vi "Create and Load SensorLUT Dictionary.vi"(8 "error in (no error)":errorcluster, 11 "Main in":refnum<class "Main.lvclass">) -> (0 "error out":errorcluster, 3 "Main out":refnum<class "Main.lvclass">)   [LabVIEW 2019, in "Main.lvclass"]
uses:
  Main.lvclass
  Main.lvclass/Main.ctl
  Common/DataTypes/Sensor LUT--cluster.ctl
  Common/DataTypes/Sensor database record--cluster.ctl
  Common/DataTypes/Sensor ranges--cluster.ctl
  Accessors/Set CurrSensor Record.vi
  Accessors/Get Settings.vi
  <userlib>/_OpenG.lib/file/file.llb/File Exists - Scalar__ogtk.vi
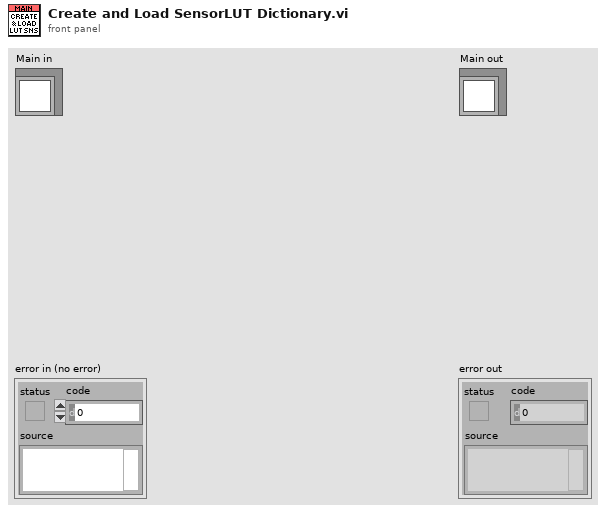
[diagram p1: front panel]
types:
  T1 = typedef "Main.lvclass/Settings--cluster.ctl" = cluster{"Simulation":bool, "Signal scaling":T2[], "ESR scaling":T3[], "num readings to average":i32[], "ESR alarm threshhold (%)":i32[], "UseDummyVrms":bool, "Dummy Vrms":dbl, "Inverter Database File":path, "default Inverter (name)":string[], "Minimum Current Threshold ":dbl[], "Sensors Database File":path, "default Sensors (name)":string[]}
  T2 = typedef "Main.lvclass/Gain control.ctl" = cluster{"Iin ripple gain":dbl, "Iout ripple gain":dbl, "Iout 60Hz gain ":dbl, "Vout 60Hz gain ":dbl, "Iin ripple offest":dbl, "Iout ripple offset":dbl, "Iout 60Hz offset":dbl, "Vout 60Hz offset":dbl}
  T3 = typedef "Main.lvclass/ESR scaling--cluster.ctl" = cluster{"Gain":dbl, "Offset":dbl}
  T4 = typedef "Sensor LUT--cluster.ctl" = T5[]
  T5 = typedef "Sensor database record--cluster.ctl" = cluster{"name":string, "last updated":timestamp, "manufacturer":string, "model":string, "Sensitivity index":dbl, "Sensor Ranges":T6}
  T6 = typedef "Sensor ranges--cluster.ctl" = cluster{"Max.VOut.RMS (V)":dbl, "Max.Out.Peak (V)":dbl, "Sensitivity (mV/A)":dbl, "Max.IOut.RMS(A)":dbl, "Min.IOut.RMS(A)":dbl}
  T7 = typedef "TD Dynamic CVT DVR--ref.ctl" = refnum<data-value>
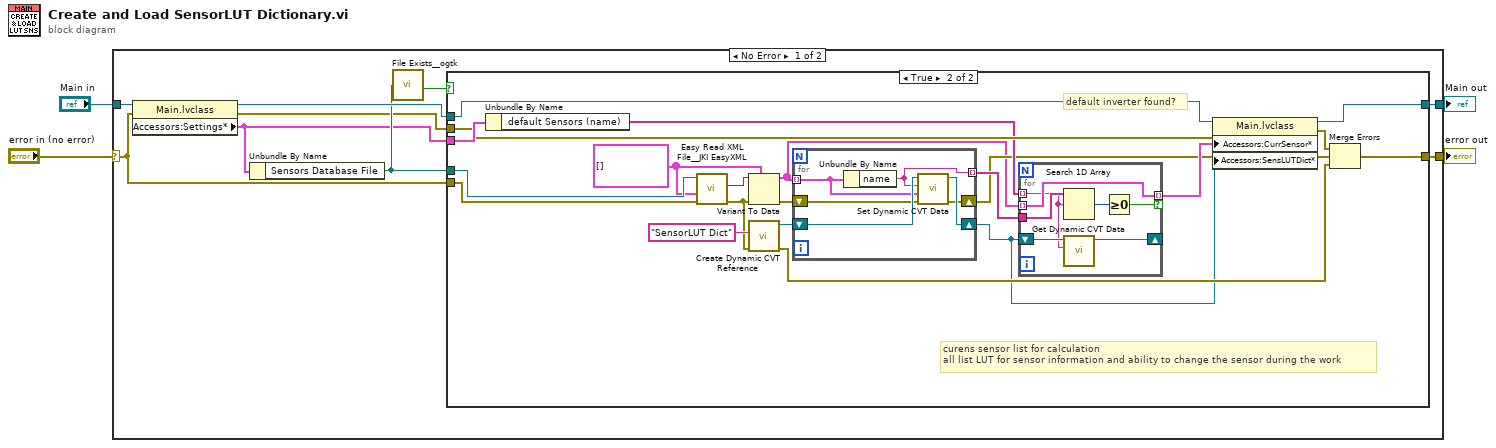
[diagram p0: block diagram]
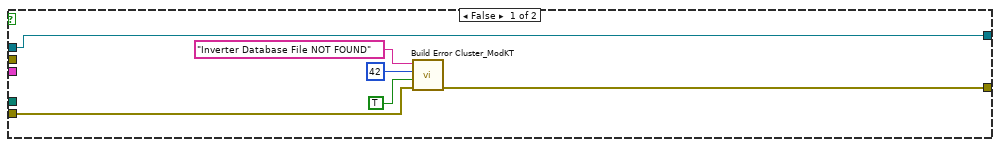
[diagram p2: hidden frame]
diagram:
  n1 = case shown="No Error" "error in (no error)" {
    selector: "error in (no error)" -> [w11 w55]
    tunnel: [w12 w55] -> w1
    tunnel: [w10 w54] -> w2
    tunnel: "Main in" -> [w13 w54]
    frame No Error {
      n2 = property class="Main.lvclass"(reference=w13, error in=w11) -> (reference out=w9:refnum<class "Main.lvclass">, error out=w5:errorcluster, "Accessors:Settings*"=w6:T1)
      n3 = Unbundle By Name(w6) -> ("Sensors Database File"=w8:path)
      n4 = call-poly <userlib>:"File Exists__ogtk.vi"("file path"=w8) -> ("exists"=w7:bool)  [unwired: 6 in, 1 out]
      n5 = case shown="True" w7 {
        tunnel: [w18 w28] -> w12
        tunnel: w8 -> [_ w38]
        tunnel: w11 -> [w17 w37]
        tunnel: [w19 w30] -> w10
        tunnel: w9 -> [w19 w36]
        tunnel: w6 -> [_ w31]
        tunnel: w5 -> [_ w29]
        frame False {
          n6 = call <vilib>:"Build Error Cluster_ModKT .vi"("Prepend String (\"\")"="Inverter Database File NOT FOUND" ("Prepend String (\"\")"), "code"=42, "error? (F)"=TRUE, "error in (no error)"=w17) -> ("error out"=w18:errorcluster)  [unwired: 3 in, 1 out]
        }
        frame True {
          w21 = T4 [] ("Sensor Records")
          # "curens sensor list for calculation\nall list LUT for sensor information and ability to change the sensor during the work"
          # "default inverter found?"
          n7 = Unbundle By Name(w31) -> ("default Sensors (name)"=w25:string[])
          n8 = call <vilib>:"Easy Read XML File__JKI EasyXML.vi"("error in (no error)"=w37, "LabVIEW Data (Type)"=w21, "XML File Path"=w38) -> ("error out"=w35:errorcluster, "LabVIEW Data"=w34:variant)  [unwired: 6 in, 1 out]
          n9 = Variant To Data(error in=w35, type=w21, Variant=w34) -> (data=w22:T4, error out=w33:errorcluster)
          n10 = call <vilib>:"Create Dynamic CVT Reference.vi"("error in (no error)"=w35, "DictName"="SensorLUT Dict") -> ("error out"=w40:errorcluster, "dCVT DVR out"=w32:T7)  [unwired: 8 in]
          n11 = for {
            tunnel: w22 -> [w49] mode=indexing
            shift-right: [w50] -> w23
            shift-left: w33 -> [w51]
            shift-right: [w52] -> w20
            shift-left: w32 -> [w53]
            tunnel: [w48] -> w26 mode=indexing
            n12 = Unbundle By Name(w49) -> ("name"=w48:string)
            n13 = call <vilib>:"Set Dynamic CVT Data.vi"("error in (no error)"=w51, "value"=w49, "DataName"=w48, "dCVT DVR"=w53) -> ("error out"=w50:errorcluster, "dCVT DVR out"=w52:T7)  [unwired: 5 in, 1 out]
          }
          n14 = for {
            tunnel: w26 -> [w47]
            tunnel: [w44] -> w24 mode=indexing if=w45
            tunnel: w22 -> [w44] mode=indexing
            tunnel: w25 -> [w41] mode=indexing
            shift-right: [w42] -> _
            shift-left: w20 -> [w43]
            n15 = Search 1D Array(1D array=w47, element=w41) -> (index of element=w46:i32)  [unwired: 1 in]
            n16 = call <vilib>:"Get Dynamic CVT Data.vi"("DataName"=w41, "dCVT DVR"=w43) -> ("dCVT DVR out"=w42:T7)  [unwired: 6 in, 3 out]
            n17 = Greater Or Equal To 0?(x=w46) -> (x >= 0?=w45:bool)
          }
          n18 = property class="Main.lvclass"(reference=w36, error in=w29, "Accessors:CurrSensor*"=w24, "Accessors:SensLUTDict*"=w20) -> (reference out=w30:refnum<class "Main.lvclass">, error out=w27:errorcluster)
          n19 = Merge Errors(w27, w23, w40) -> (w28:errorcluster)
        }
      }
    }
    frame Error {
    }
  }
  "error out" <- w1
  "Main out" <- w2
